vi "7HP_Close serial port.vi"(8 "Error in":errorcluster, 11 "VISA resource name":refnum<visa-resource-name>) -> (0 "Error out":errorcluster)   [LabVIEW 2021]
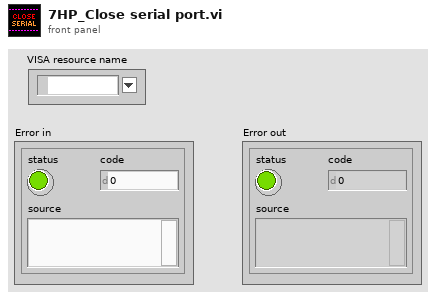
[diagram p1: front panel]
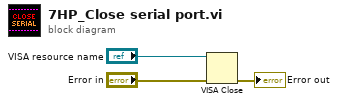
[diagram p0: block diagram]
diagram:
  n1 = VISA Close(VISA resource name="VISA resource name", error in (no error)="Error in") -> (error out=→"Error out":errorcluster)
